vi "Prime BSI Camera Engine.vi"(0 "Prime Notifier Name":string="Not a Name", 11 "Camera Index":string[](array[string])) -> ()   [LabVIEW 2016]
uses:
  Prime BSI Controls/Prime Parameters.ctl
  Prime BSI Controls/Prime Parameter List.ctl
  Prime BSI Controls/Prime ROI.ctl
  Prime BSI Controls/Prime Notifier Element.ctl
  Prime BSI Controls/Prime Actions.ctl
  <vilib>/vision/Image Controls.llb/IMAQ Image.ctl
  Prime BSI Controls/Prime IMAQ Key Info.ctl
  TIFF Image Read and Write/TIF Write Image Information.ctl
  <vilib>/ptbypt/NI_PtbyPt.lvlib
panel:
  in  "Timing Mode":u32=1
  in  "Set Trigger":bool
  out "mean":dbl format="%0.2f"
  out "Value":dbl format="%.2f"
  in  "Parameter ID":u32
  out "fps":dbl
  out "Image Key Error":errorcluster
  out "Frame":u32
  in  "Init Camera":bool
  in  "Quit":bool
  in  "Use Display Module":bool
  in  "Capture":bool
  in  "Live Preview":bool
  in  "Get ROI":bool
  in  "Set ROI":bool
  in  "Get Parameter":bool
  in  "Set Parameter":bool
  in  "File Save Path":path
  in  "# of Frames":u32
  in  "ROI Setup":T1
  in  "Prime Parameter":T2
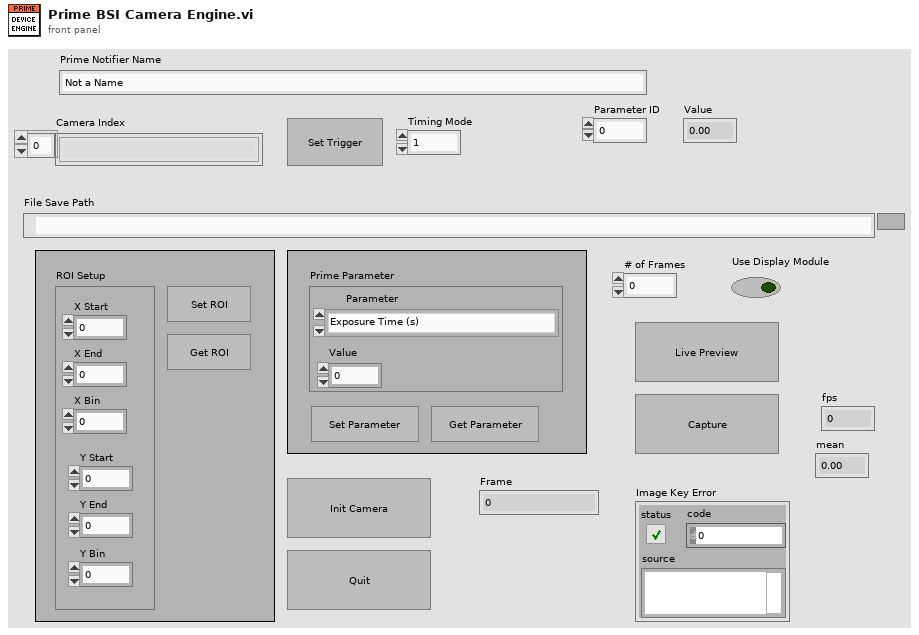
[diagram p1: front panel]
types:
  T1 = typedef "Prime ROI.ctl" = cluster{"X Start":u32, "X End":u32, "X Bin":u32, "Y Start":u32, "Y End":u32, "Y Bin":u32}
  T2 = typedef "Prime Parameters.ctl" = cluster{"Parameter":T3, "Value":dbl}
  T3 = typedef "Prime Parameter List.ctl" = enum16{"Exposure Time (s)"}
  T4 = typedef "Prime Actions.ctl" = enum16{"Error Check", "Initialize", "Preview", "Record", "Abort", "Record Settings", "Set Parameter", "Get Parameter", "Set ROI", "Get ROI", "Status", "Set Trigger", "Quit"}
  T5 = typedef "Image Type" = u32
  T6 = typedef "Prime Notifier Element.ctl" = cluster{"Prime Actions":T4, "Received?":bool, "Prime Parameter":T2, "Prime ROI":T1, "Running?":bool, "File Path":path, "# of frames":u32, "Image Ref":T7, "Error":errorcluster}
  T7 = typedef "IMAQ Image.ctl" = refnum<image>
  T8 = typedef "Prime IMAQ Key Info.ctl" = cluster{"Frame":u32, "Sensor Height":i32, "Sensor Width":i32, "ROI Height":i32, "ROI Width":i32, "ROI Enable?":bool, "Bit per Pixel":u8}
  T9 = enum32{"Invalid", "Standard", "Closed", "Hidden", "Minimized", "Maximized"}
  T10 = typedef "TIF Write Image Information.ctl" = cluster{"Image Width (Pixels)":u32, "Image Height (Pixels)":u32, "Pixel Width (µm)":dbl, "Pixel Height (µm)":dbl, "Bits Per Sample (e.g. 16)":u32, "No. of Frames":u32, "No. of Slices":u32, "Time Step (sec)":dbl, "Z Step (µm)":dbl}
  T11 = enum16{"big-endian, network order", "native, host order", "little-endian"}
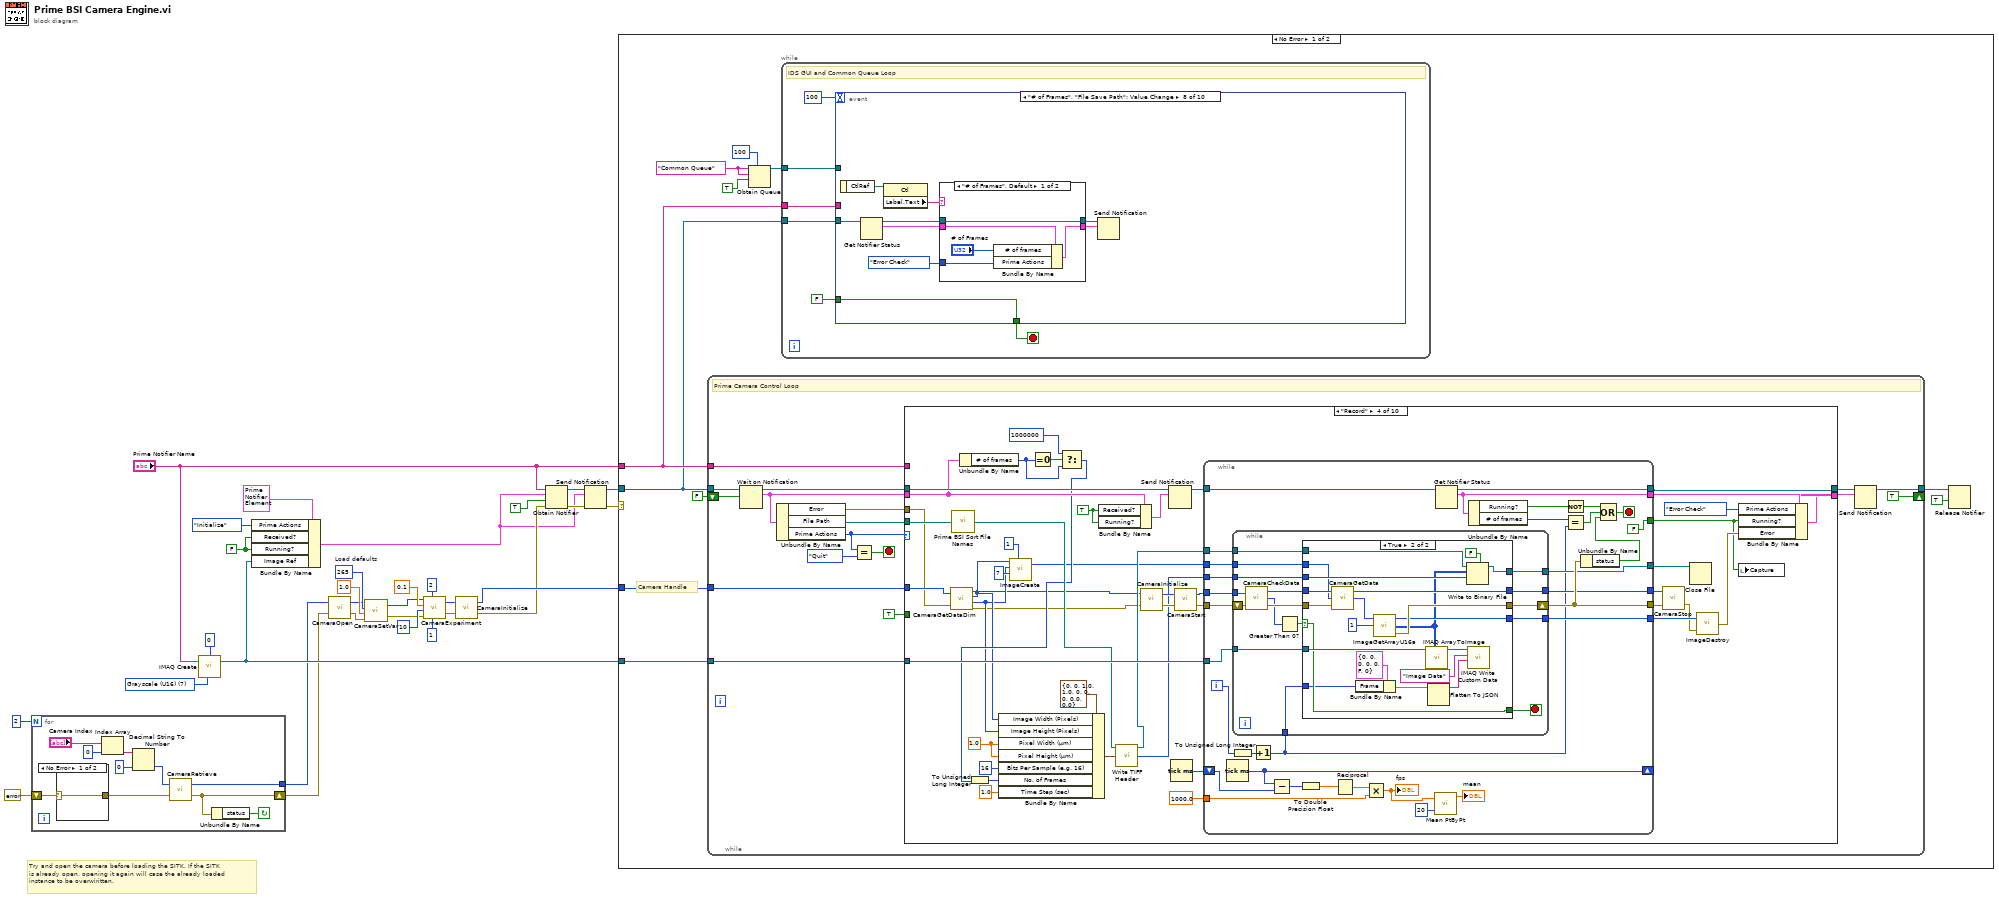
[diagram p0: block diagram]
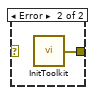
[diagram p2: hidden frame]
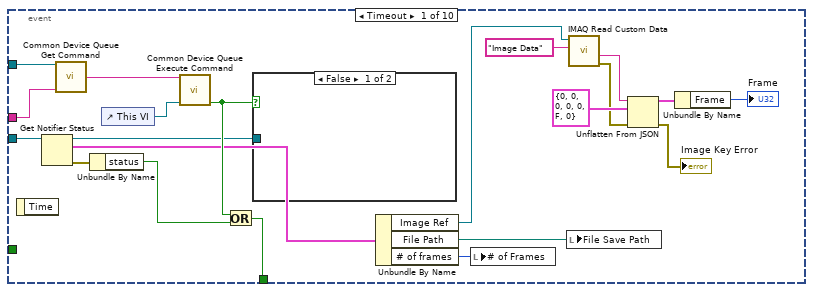
[diagram p3: hidden frame]
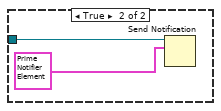
[diagram p4: hidden frame]
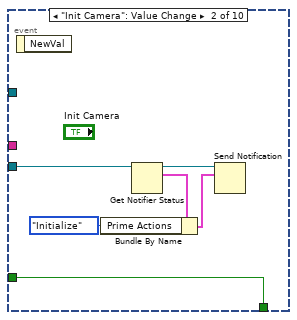
[diagram p5: hidden frame]
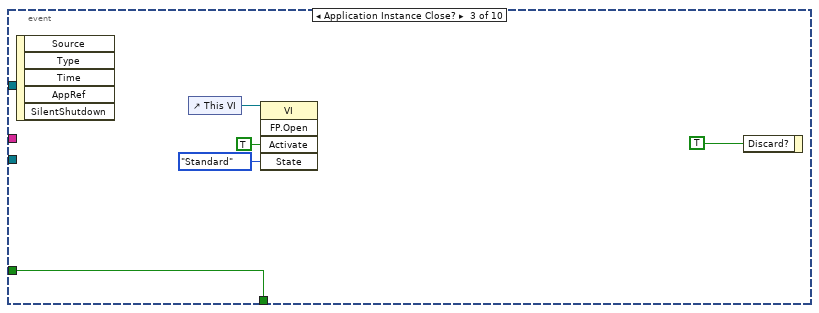
[diagram p6: hidden frame]
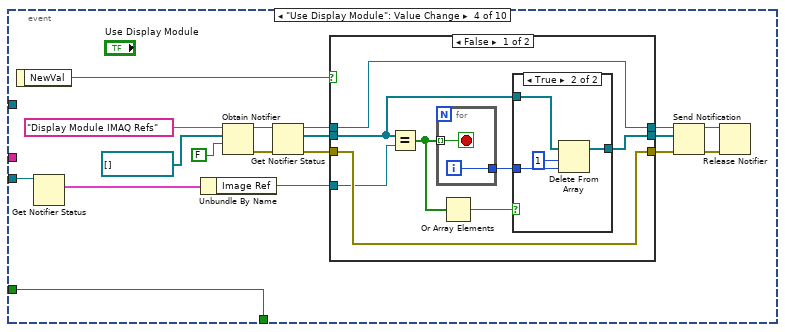
[diagram p7: hidden frame]
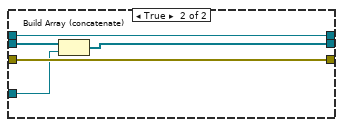
[diagram p9: hidden frame]
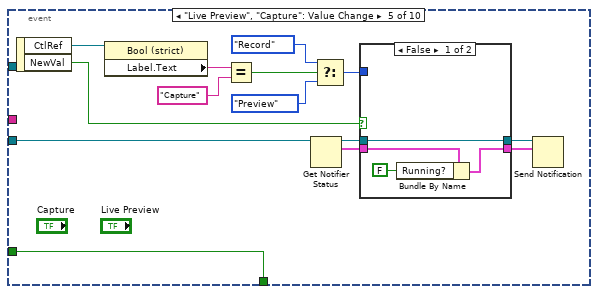
[diagram p10: hidden frame]
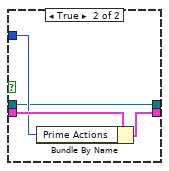
[diagram p11: hidden frame]
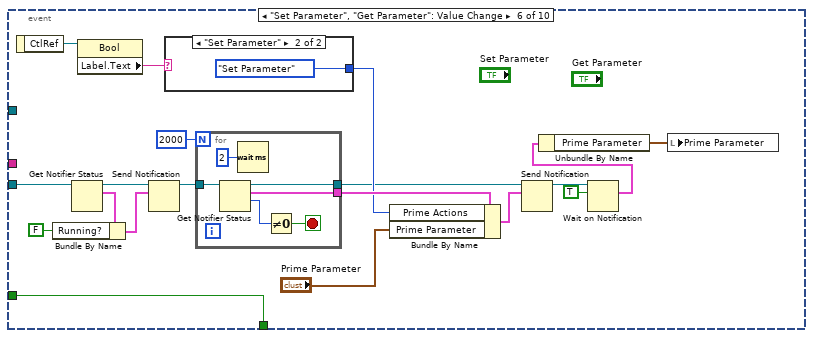
[diagram p12: hidden frame]
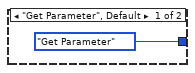
[diagram p13: hidden frame]
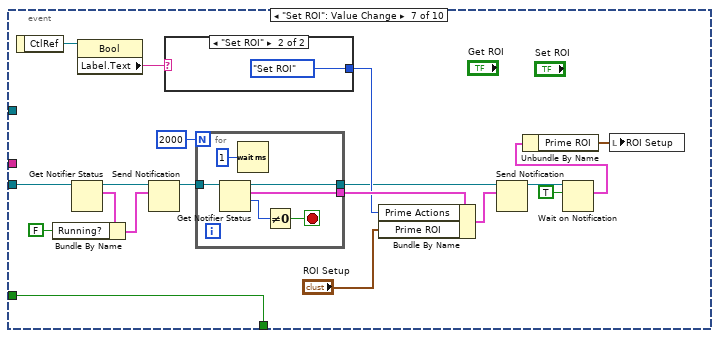
[diagram p14: hidden frame]
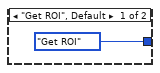
[diagram p15: hidden frame]
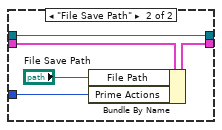
[diagram p16: hidden frame]
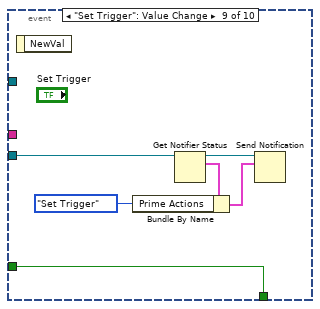
[diagram p17: hidden frame]
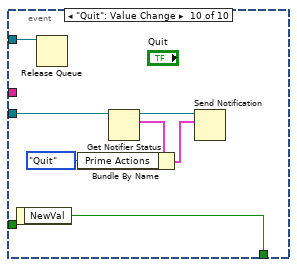
[diagram p18: hidden frame]
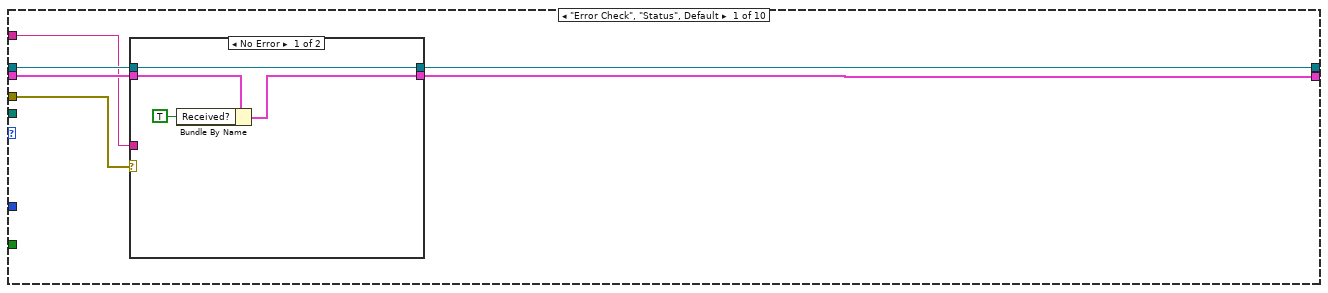
[diagram p19: hidden frame]
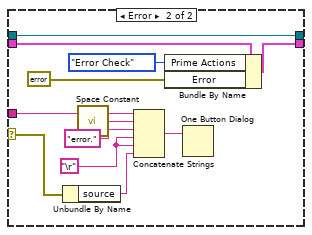
[diagram p20: hidden frame]
diagram:
  w19 = u32 265  # Load defaults
  w21 = FALSE ("Received?")
  w25 = T5 7 items=["Grayscale (U8)", "Grayscale (I16)", "Grayscale (SGL)", "Complex (CSG)", "RGB (U32)", "HSL (U32)", "RGB (U64)", "Grayscale (U16)"] ("Image Type")
  # "Try and open the camera before loading the SITK. If the SITK\nis already open, opening it again will case the already loaded\ninstance to be overwiritten."
  n1 = for {
    N: 2 -> [_]
    tunnel: [w36] -> w13
    shift-right: [w33] -> w12
    shift-left: errorcluster {"status"=FALSE, "code"=0, "source"=""} ("error out") -> [w35]
    stop <- w32 continue-if-true
    n2 = case shown="No Error" w35 {
      selector: w35 -> [w42 _]
      tunnel: [w42 w43] -> w34
      frame No Error {
      }
      frame Error {
        n3 = call <userlib>:"InitToolkit.vi"() -> ("error out"=w43:errorcluster)  [unwired: 1 in]
      }
    }
    n4 = Index Array(array="Camera Index", index=0) -> (element=w39:string)
    n5 = Decimal String To Number(string=w39, default (0L)=u32 0 ("default (0 I32)")) -> (number=w37:u32)  [unwired: 1 in, 1 out]
    n6 = call <userlib>:"CameraRetrieve.vi"("error in"=w34, "Camera Index"=w37) -> ("error out"=w33:errorcluster, "Device ID"=w36:u32)
    n7 = Unbundle By Name(w33) -> ("status"=w32:bool)
  }
  n8 = call "IMAQ Create"("Border Size"=0, "Image Name"="Prime Notifier Name", "Image Type"=w25) -> ("New Image"=w20:T7)  [unwired: 2 in, 1 out]
  n9 = Bundle By Name(cluster=T6 {"Prime Actions"=enum."Initialize", "Received?"=FALSE, "Prime Parameter"={"Parameter"=enum."Exposure Time (s)", "Value"=0.0}, "Prime ROI"={"X Start"=0, "X End"=0, "X Bin"=0, "Y Start"=0, "Y End"=0, "Y Bin"=0}, "Running?"=FALSE, "File Path"=path "", "# of frames"=0, "Image Ref"=refnum, "Error"={"status"=FALSE, "code"=0, "source"=""}} ("IDS Camera Cluster"), "Prime Actions"=Prime_Actions."Initialize" ("IDS Actions"), "Received?"=w21, "Running?"=w21, "Image Ref"=w20) -> (w1:T6)
  n10 = call <userlib>:"CameraOpen.vi"("error in"=w12, "Camera Device ID"=w13) -> ("error out"=w17:errorcluster, "Camera Handle"=w16:u32)
  n11 = call <userlib>:"CameraSetVar.vi"("error in"=w17, "Value"=1.0, "Parameter ID"=w19, "Camera Handle"=w16) -> ("error out"=w4:errorcluster, "CameraHandle"=w5:u32)
  n12 = call <userlib>:"CameraExperiment.vi"("Number of Accumulations"=u32 1, "Acquire / Focus Flag"=u32 2, "error in"=w4, "Number of Images"=u32 10 ("Acquire / Focus Flag"), "Exposure (sec)"=0.1, "Camera Handle"=w5) -> ("error out"=w10:errorcluster, "Camera Handle"=w11:u32)
  n13 = call <userlib>:"CameraInitialize.vi"("error in"=w10, "Camera Handle"=w11) -> ("error out"=w2:errorcluster, "Camera Handle"=w3:u32)
  n14 = Obtain Notifier(name (unnamed)="Prime Notifier Name", notification data type=w1, create if not found? (T)=TRUE, error in (no error)=w2) -> (notifier out=w30:refnum<notifier>, error out=w29:errorcluster)  [unwired: 1 out]
  n15 = Send Notification(notification=w1, notifier=w30, error in (no error)=w29) -> (notifier out=w28:refnum<notifier>, error out=w27:errorcluster)
  n16 = case shown="No Error" w27 {
    selector: w27 -> [_ w603]
    tunnel: w28 -> [w45 w604]
    tunnel: "Prime Notifier Name" -> [w46 w602]
    tunnel: w3 -> [w44 w593]
    tunnel: w20 -> [w52 w596]
    frame No Error {
      w50 = "Common Queue" ("Unique Notifier Name")
      # "Camera Handle"
      n17 = while {
        tunnel: w45 -> [w255]
        tunnel: [w256] -> w53
        tunnel: w44 -> [w249]
        tunnel: w52 -> [w248]
        tunnel: w46 -> [w244]
        shift-right: [TRUE] -> _
        shift-left: FALSE -> [w247]
        stop <- w257 stop-if-true
        # "Prime Camera Control Loop"
        n18 = Wait on Notification(notifier=w255, ignore previous (F)=w247) -> (notifier out=w254:refnum<notifier>, notification=w253:T6)  [unwired: 2 in, 2 out]
        n19 = Unbundle By Name(w253) -> ("Error"=w243:errorcluster, "File Path"=w241:path, "Prime Actions"=w252:T4)
        n20 = Equal?(x=w252, y=Prime_Actions."Quit") -> (x = y?=w257:bool)
        n21 = case shown="\"Record\"" w252 {
          tunnel: w254 -> [w263 w326 w355 w443 w518 w535 w547 w569 w582 w590]
          tunnel: [w262 w326 w334 w428 w518 w535 w547 w569 w582 w590] -> w250
          tunnel: w253 -> [w261 w325 w354 w417 w519 w533 w548 w570 w580 w589]
          tunnel: w244 -> [w260 _ _ _ _ _ _ _ _ _]
          tunnel: w249 -> [_ w312 w349 w438 w522 w530 w564 _ w576 w584]
          tunnel: w248 -> [_ w281 w340 w433 _ _ w551 _ _ w586]
          tunnel: [w259 w323 w353 w442 w525 w536 w566 w572 w578 w587] -> w246
          tunnel: TRUE -> [_ _ _ _ _ _ _ _ _ _]
          tunnel: w243 -> [w258 w280 w327 w398 w523 _ w546 w571 _ _]
          tunnel: w241 -> [_ _ _ w423 _ _ _ _ _ _]
          frame "Error Check", "Status", Default {
            n22 = case shown="No Error" w258 {
              selector: w258 -> [_ w270]
              tunnel: w261 -> [w266 w279]
              tunnel: [w267 w277] -> w262
              tunnel: w263 -> [w267 w277]
              tunnel: w260 -> [_ w276]
              tunnel: [w264 w272] -> w259
              frame No Error {
                n23 = Bundle By Name(cluster=w266, "Received?"=TRUE) -> (w264:T6)
              }
              frame Error {
                w271 = "\r"
                n24 = Unbundle By Name(w270) -> ("source"=w269:string)
                n25 = call <vilib>:"Space Constant.vi"() -> ("String"=w275:string)
                n26 = Concatenate Strings(w276, w275, "error." ("string"), w271, w271, w269) -> (w273:string)
                n27 = Bundle By Name(cluster=w279, "Prime Actions"=Prime_Actions."Error Check" ("IDS Actions"), "Error"=errorcluster {"status"=FALSE, "code"=0, "source"=""}) -> (w272:T6)
                n28 = One Button Dialog(message=w273) -> ()  [unwired: 1 in, 1 out]
              }
            }
          }
          frame "Initialize" {
            w287 = -2  # -2 = fastest adc
            w283 = -1  # -1 = keep what is currently set
            w291 = u32 1 items=["N/A", "Timed Mode/Free run", "Trigger First (only PM)", "Strobed/Ext Sync"] ("Timing Mode")
            w290 = u32 2  # Trigger Edge
            w295 = u32 3  # Shutter State
            w294 = u32 0  # Shutter Comp Time
            w299 = u32 1  # Number of Clears
            w298 = u32 50  # Number of Strips Per Clear
            w300 = u32 0  # Continuous Clears
            w282 = u32 2048 ("X End")
            w304 = u32 1 ("X Start")
            w306 = u32 1  # ROI Number
            w309 = u32 2 items=["Never", "Pre Expos", "Pre Seq", "Post Seq", "Pre-Post Seq", "Pre Expos, Post Seq"] ("Clear Mode")
            w310 = u32 32  # Clear Mode
            w313 = u32 0 items=["First Row", "All Rows", "Any Row", "Max Exposure"] ("Exposure Out")
            w315 = u32 255  # Exposure Out
            n29 = To Double Precision Float(number=w313) -> (double precision float=w314:dbl)
            n30 = call <userlib>:"CameraSetVar.vi"("error in"=w280, "Value"=w314, "Parameter ID"=w315, "Camera Handle"=w312) -> ("error out"=w307:errorcluster, "CameraHandle"=w308:u32)
            n31 = To Double Precision Float(number=w309) -> (double precision float=w311:dbl)
            n32 = Bundle By Name(cluster=T1 {"X Start"=0, "X End"=0, "X Bin"=0, "Y Start"=0, "Y End"=0, "Y Bin"=0} ("ROI Setup"), "X Start"=w304, "X End"=w282, "X Bin"=w304, "Y Start"=w304, "Y End"=w282, "Y Bin"=w304) -> (w303:T1)
            n33 = call <userlib>:"CameraSetVar.vi"("error in"=w307, "Value"=w311, "Parameter ID"=w310, "Camera Handle"=w308) -> ("error out"=w301:errorcluster, "CameraHandle"=w302:u32)
            n34 = call <userlib>:"CameraROI.vi"("error in"=w301, "ROI Params"=w303, "ROI Index"=w306, "Camera Handle"=w302) -> ("error out"=w296:errorcluster, "Camera Handle"=w297:u32)
            n35 = Bundle By Name(cluster=T8 {"Frame"=0, "Sensor Height"=0, "Sensor Width"=0, "ROI Height"=0, "ROI Width"=0, "ROI Enable?"=FALSE, "Bit per Pixel"=0} ("IDS IMAQ Key Info"), "Frame"=u32 0, "Sensor Height"=w282, "Sensor Width"=w282, "ROI Height"=w282, "ROI Width"=w282, "ROI Enable?"=FALSE, "Bit per Pixel"=u8 16) -> (w320:T8)
            n36 = call <userlib>:"CameraCleans.vi"("Camera Handle"=w297, "Number of Clears"=w299, "Number of Strips Per Clear"=w298, "error in"=w296, "Continuous Clears"=w300) -> ("Camera Handle"=w293:u32, "error out"=w292:errorcluster)
            n37 = call <userlib>:"CameraShutter.vi"("Camera Handle"=w293, "Shutter Comp Time: Pre Open"=w294, "Shutter Comp Time: Post Open"=w294, "error in"=w292, "Shutter State"=w295) -> ("Camera Handle"=w289:u32, "error out"=w288:errorcluster)
            n38 = Flatten To JSON(anything=w320) -> (JSON string=w322:string)  [unwired: 2 in, 1 out]
            n39 = call <userlib>:"CameraTrigger.vi"("error in"=w288, "Trigger Edge"=w290, "Timing Mode"=w291, "Camera Handle"=w289) -> ("error out"=w285:errorcluster, "Camera Handle"=w286:u32)
            n40 = call "IMAQ Write Custom Data"("Custom Data In"=w322, "Key"="Image Data", "Image"=w281) -> ()  [unwired: 7 in, 2 out]
            n41 = call <userlib>:"CameraADCset.vi"("ADC offset"=w283, "Read Out port"=w283, "error in (no error)"=w285, "ADC Gain"=w283, "ADC Speed"=w287, "Camera Handle"=w286) -> ("error out"=w284:errorcluster)  [unwired: 1 out]
            n42 = Bundle By Name(cluster=w325, "Prime Actions"=Prime_Actions."Error Check" ("IDS Actions"), "Error"=w284) -> (w323:T6)
          }
          frame "Preview" {
            w331 = FALSE ("Running?")
            w351 = TRUE ("Received?")
            n43 = Bundle By Name(cluster=w354, "Received?"=w351, "Running?"=w351) -> (w352:T6)
            n44 = call <userlib>:"CameraGetDataDim.vi"("Camera Handle"=w349, "error in"=w327) -> ("Camera Handle"=w329:u32, "Xdim"=w348:u32, "Ydim"=w347:u32, "error out"=w344:errorcluster)
            n45 = call <userlib>:"ImageCreate.vi"("X dimension"=w348, "Y dimension"=w347, "Data Type"=u32 7, "error in"=w344, "Number Of Frames"=u32 1) -> ("Image Handle"=w343:u32, "error out"=w328:errorcluster)
            n46 = Send Notification(notification=w352, notifier=w355) -> (notifier out=w339:refnum<notifier>)  [unwired: 1 in, 1 out]
            n47 = call <userlib>:"CameraStart.vi"("error in"=w328, "Camera Handle"=w329) -> ("error out"=w341:errorcluster, "Camera Handle"=w342:u32)
            n48 = while {
              tunnel: w342 -> [w375]
              tunnel: w341 -> [w374]
              tunnel: w343 -> [w371]
              tunnel: w339 -> [w361]
              tunnel: [w360] -> w334
              tunnel: [w363] -> w336
              tunnel: [w373] -> w337
              tunnel: [w372] -> w335
              tunnel: w340 -> [w370]
              tunnel: [w358] -> w333
              shift-right: [w356] -> _
              shift-left: u32 0 ("Frame") -> [w357]
              stop <- w369 stop-if-true
              n49 = call <userlib>:"CameraCheckData.vi"("Camera Handle"=w375, "error in"=w374) -> ("Camera Handle"=w367:u32, "Number Of Frames Available"=w365:i32, "error out"=w368:errorcluster)
              n50 = Greater Than 0?(x=w365) -> (x > 0?=w366:bool)
              n51 = case shown="True" w366 {
                tunnel: w371 -> [w377 w394]
                tunnel: w368 -> [w379 w392]
                tunnel: [w379 w397] -> w363
                tunnel: [w377 w396] -> w372
                tunnel: [w378 w390] -> w373
                tunnel: w367 -> [w378 w393]
                tunnel: w370 -> [_ w387]
                tunnel: w357 -> [w376 w381]
                tunnel: [w376 w380] -> w356
                frame False {
                }
                frame True {
                  n52 = Increment(x=w381) -> (x+1=w380:u32)
                  n53 = call <userlib>:"CameraGetData.vi"("error in"=w392, "Image/Data Handle"=w394, "Camera Handle"=w393) -> ("error out"=w389:errorcluster, "Image/Data Handle"=w391:u32, "Camera Handle"=w390:u32)
                  n54 = Bundle By Name(cluster=T8 {"Frame"=0, "Sensor Height"=0, "Sensor Width"=0, "ROI Height"=0, "ROI Width"=0, "ROI Enable?"=FALSE, "Bit per Pixel"=0} ("IDS IMAQ Key Info"), "Frame"=w380) -> (w383:T8)
                  n55 = call <userlib>:"ImageGetArrayU16a.vi"("error in"=w389, "Z position"=u32 1, "Data Handle"=w391) -> ("error out"=w397:errorcluster, "Array uint 16"=w388:u16[][], "Data Handle"=w396:u32)  [unwired: 1 in]
                  n56 = call "IMAQ ArrayToImage"("Image Pixels (U16)"=w388, "Image"=w387) -> ("Image Out"=w382:T7)  [unwired: 8 in, 1 out]
                  n57 = Flatten To JSON(anything=w383) -> (JSON string=w385:string)  [unwired: 2 in, 1 out]
                  n58 = call "IMAQ Write Custom Data"("Custom Data In"=w385, "Key"="Image Data", "Image"=w382) -> ()  [unwired: 7 in, 2 out]
                }
              }
              n59 = Get Notifier Status(notifier=w361) -> (notifier out=w360:refnum<notifier>, current notification=w358:T6)  [unwired: 1 in, 3 out]
              n60 = Unbundle By Name(w358) -> ("Running?"=w362:bool)
              n61 = Unbundle By Name(w363) -> ("status"=w364:bool)
              n62 = Not(x=w362) -> (.not. x?=w359:bool)
              n63 = Or(x=w359, y=w364) -> (x .or. y?=w369:bool)
            }
            n64 = call <userlib>:"CameraStop.vi"("error in"=w336, "Camera Handle"=w337) -> ("error out"=w338:errorcluster)  [unwired: 1 out]
            n65 = call <userlib>:"ImageDestroy.vi"("error in"=w338, "Data handle"=w335) -> ("error out"=w332:errorcluster)
            n66 = Bundle By Name(cluster=w333, "Prime Actions"=Prime_Actions."Error Check", "Running?"=w331, "Error"=w332) -> (w353:T6)
            n67 = local write "Capture"(w331) -> ()
          }
          frame "Record" {
            w420 = 1.0 ("Pixel Width (µm)")
            w440 = TRUE ("Received?")
            n68 = call <userlib>:"CameraGetDataDim.vi"("Camera Handle"=w438, "error in"=w398) -> ("Camera Handle"=w400:u32, "Xdim"=w406:u32, "Ydim"=w405:u32, "error out"=w399:errorcluster)
            n69 = call "Prime BSI Sort File Names.vi"("Requested File Path"=w423) -> ("Resulting File Path"=w418:path)  [unwired: 14 in]
            n70 = Unbundle By Name(w417) -> ("# of frames"=w415:u32)
            n71 = call <userlib>:"ImageCreate.vi"("X dimension"=w406, "Y dimension"=w405, "Data Type"=u32 7, "Number Of Frames"=u32 1) -> ("Image Handle"=w404:u32)  [unwired: 1 in, 1 out]
            n72 = Equal To 0?(x=w415) -> (x = 0?=w416:bool)
            n73 = Select(t=1000000, s=w416, f=w415) -> (s? t:f=w413:u32)
            n74 = To Unsigned Long Integer(number=w413) -> (unsigned 32bit integer=w403:u32)
            n75 = Bundle By Name(cluster=T10 {"Image Width (Pixels)"=0, "Image Height (Pixels)"=0, "Pixel Width (µm)"=1.0, "Pixel Height (µm)"=1.0, "Bits Per Sample (e.g. 16)"=0, "No. of Frames"=0, "No. of Slices"=0, "Time Step (sec)"=0.0, "Z Step (µm)"=0.0} ("Image Info"), "Image Width (Pixels)"=w406, "Image Height (Pixels)"=w405, "Pixel Width (µm)"=w420, "Pixel Height (µm)"=w420, "Bits Per Sample (e.g. 16)"=u32 16, "No. of Frames"=w403, "Time Step (sec)"=1.0) -> (w422:T10)
            n76 = Bundle By Name(cluster=w417, "Received?"=w440, "Running?"=w440) -> (w441:T6)
            n77 = call "Write TIFF Header.vi"("File Path"=w418, "Image Info"=w422) -> ("File Ref"=w411:refnum<file>, "Byte Order"=w410:T11)  [unwired: 11 in, 1 out]
            n78 = call <userlib>:"CameraInitialize.vi"("error in"=w399, "Camera Handle"=w400) -> ("error out"=w437:errorcluster, "Camera Handle"=w436:u32)
            n79 = Send Notification(notification=w441, notifier=w443) -> (notifier out=w432:refnum<notifier>)  [unwired: 1 in, 1 out]
            n80 = Tick Count (ms)() -> (millisecond timer value=w425:u32)
            n81 = call <userlib>:"CameraStart.vi"("error in"=w437, "Camera Handle"=w436) -> ("error out"=w434:errorcluster, "Camera Handle"=w435:u32)
            n82 = while {
              tunnel: w435 -> [w475]
              tunnel: w434 -> [w474]
              tunnel: w432 -> [w473]
              tunnel: [w472] -> w428
              tunnel: [w469] -> w430
              tunnel: [w468] -> w431
              tunnel: [w467] -> w429
              tunnel: w433 -> [w465]
              tunnel: [w464] -> w427
              shift-right: [w458] -> _
              shift-left: w425 -> [w459]
              tunnel: 1000.0 -> [w454]
              tunnel: w411 -> [w453]
              tunnel: w410 -> [w452]
              tunnel: [w451] -> w409
              tunnel: w404 -> [w450]
              tunnel: [FALSE ("Running?")] -> w402
              i -> [w462]
              stop <- w470 stop-if-true
              n83 = Tick Count (ms)() -> (millisecond timer value=w458:u32)
              n84 = To Unsigned Long Integer(number=w462) -> (unsigned 32bit integer=w444:u32)
              n85 = Increment(x=w444) -> (x+1=w448:u32)
              n86 = while {
                tunnel: w475 -> [w491]
                tunnel: [w486] -> w468
                tunnel: [w485] -> w467
                tunnel: w465 -> [w482]
                shift-right: [w488] -> w469
                shift-left: w474 -> [w490]
                tunnel: w453 -> [w480]
                tunnel: w452 -> [w479]
                tunnel: [w478] -> w451
                tunnel: w450 -> [w477]
                tunnel: w448 -> [w476]
                stop <- w481 stop-if-true
                n87 = call <userlib>:"CameraCheckData.vi"("Camera Handle"=w491, "error in"=w490) -> ("Camera Handle"=w487:u32, "Number Of Frames Available"=w484:i32, "error out"=w489:errorcluster)
                n88 = Greater Than 0?(x=w484) -> (x > 0?=w483:bool)
                n89 = case shown="True" w483 {
                  selector: w483 -> [w494 w505]
                  tunnel: w489 -> [w496 w513]
                  tunnel: [w496 w517] -> w488
                  tunnel: [w492 w516] -> w485
                  tunnel: [w495 w512] -> w486
                  tunnel: w487 -> [w495 w514]
                  tunnel: w482 -> [_ w511]
                  tunnel: w476 -> [_ w497]
                  tunnel: [w494 w505] -> w481
                  tunnel: w480 -> [w493 w502]
                  tunnel: w479 -> [_ w501]
                  tunnel: [w493 w499] -> w478
                  tunnel: w477 -> [w492 w498]
                  frame False {
                  }
                  frame True {
                    n90 = call <userlib>:"CameraGetData.vi"("error in"=w513, "Image/Data Handle"=w498, "Camera Handle"=w514) -> ("Image/Data Handle"=w504:u32, "Camera Handle"=w512:u32)  [unwired: 1 out]
                    n91 = Bundle By Name(cluster=T8 {"Frame"=0, "Sensor Height"=0, "Sensor Width"=0, "ROI Height"=0, "ROI Width"=0, "ROI Enable?"=FALSE, "Bit per Pixel"=0} ("IDS IMAQ Key Info"), "Frame"=w497) -> (w507:T8)
                    n92 = call <userlib>:"ImageGetArrayU16a.vi"("Z position"=u32 1, "Data Handle"=w504) -> ("error out"=w517:errorcluster, "Array uint 16"=w500:u16[][], "Data Handle"=w516:u32)  [unwired: 2 in]
                    n93 = call "IMAQ ArrayToImage"("Image Pixels (U16)"=w500, "Image"=w511) -> ("Image Out"=w506:T7)  [unwired: 8 in, 1 out]
                    n94 = Flatten To JSON(anything=w507) -> (JSON string=w509:string)  [unwired: 2 in, 1 out]
                    n95 = Write to Binary File(file (use dialog)=w502, data=w500, 5:FALSE ("prepend array or string size? (T)"), 9:w501) -> (refnum out=w499:refnum<file>)  [unwired: 2 in, 2 out]
                    n96 = call "IMAQ Write Custom Data"("Custom Data In"=w509, "Key"="Image Data", "Image"=w506) -> ()  [unwired: 7 in, 2 out]
                  }
                }
              }
              n97 = Subtract(x=w458, y=w459) -> (x-y=w457:u32)
              n98 = To Double Precision Float(number=w457) -> (double precision float=w456:dbl)
              n99 = Reciprocal(x=w456) -> (1/x=w455:dbl)
              n100 = Multiply(x=w455, y=w454) -> (x*y=w447:dbl)
              "fps" <- w447
              n101 = call <vilib>:"Mean PtByPt.vi"("x"=w447, "sample length"=20) -> ("mean"=→"mean":dbl)  [unwired: 2 in, 1 out]
              n102 = Get Notifier Status(notifier=w473) -> (notifier out=w472:refnum<notifier>, current notification=w464:T6)  [unwired: 1 in, 3 out]
              n103 = Unbundle By Name(w464) -> ("Running?"=w471:bool, "# of frames"=w463:u32)
              n104 = Not(x=w471) -> (.not. x?=w466:bool)
              n105 = Equal?(x=w463, y=w448) -> (x = y?=w461:bool)
              n106 = Unbundle By Name(w469) -> ("status"=w460:bool)
              n107 = Compound Arithmetic op=OR(w466, w461, w460) -> (w470:bool)
            }
            n108 = call <userlib>:"CameraStop.vi"("error in"=w430, "Camera Handle"=w431) -> ("error out"=w412:errorcluster)  [unwired: 1 out]
            n109 = Close File(refnum=w409) -> ()  [unwired: 1 in, 2 out]
            n110 = call <userlib>:"ImageDestroy.vi"("error in"=w412, "Data handle"=w429) -> ("error out"=w426:errorcluster)
            n111 = Bundle By Name(cluster=w427, "Prime Actions"=Prime_Actions."Error Check", "Running?"=w402, "Error"=w426) -> (w442:T6)
            n112 = local write "Capture"(w402) -> ()
          }
          frame "Get Parameter" {
            n113 = call <userlib>:"CameraGetVar.vi"("Parameter ID"="Parameter ID", "Camera Handle"=w522) -> ("Value"=→"Value":dbl)  [unwired: 1 in, 2 out]
            n114 = Bundle By Name(cluster=w519, "Prime Actions"=Prime_Actions."Error Check" ("IDS Actions"), "Error"=w523, "Received?"=TRUE) -> (w525:T6)
          }
          frame "Set Parameter" {
            n115 = Unbundle By Name(w533) -> ("Prime Parameter.Parameter"=w532:T3, "Prime Parameter.Value"=w531:dbl)
            n116 = case shown="\"Exposure Time (s)\", Default" w532 {
              tunnel: w531 -> [w541]
              tunnel: [w540] -> w529
              tunnel: w530 -> [w539]
              tunnel: [w538] -> w528
              frame "Exposure Time (s)", Default {
                n117 = call <userlib>:"CameraExperiment.vi"("Number of Accumulations"=u32 1, "Acquire / Focus Flag"=u32 2, "Number of Images"=u32 10 ("Acquire / Focus Flag"), "Exposure (sec)"=w541, "Camera Handle"=w539) -> ("error out"=w540:errorcluster, "Camera Handle"=w538:u32)  [unwired: 1 in]
              }
            }
            n118 = call <userlib>:"CameraInitialize.vi"("error in"=w529, "Camera Handle"=w528) -> ("error out"=w527:errorcluster)  [unwired: 1 out]
            n119 = Bundle By Name(cluster=w533, "Prime Actions"=Prime_Actions."Error Check" ("IDS Actions"), "Received?"=TRUE, "Error"=w527) -> (w536:T6)
          }
          frame "Set ROI" {
            w552 = "Image Data" ("Key")
            n120 = Unbundle By Name(w548) -> ("Prime ROI"=w563:T1)
            n121 = call <userlib>:"CameraROI.vi"("error in"=w546, "ROI Params"=w563, "ROI Index"=u32 1, "Camera Handle"=w564) -> ("error out"=w561:errorcluster, "Camera Handle"=w562:u32)
            n122 = call <userlib>:"CameraGetDataDim.vi"("Camera Handle"=w562, "error in"=w561) -> ("Xdim"=w550:u32, "Ydim"=w549:u32, "error out"=w545:errorcluster)  [unwired: 1 out]
            n123 = Bundle By Name(cluster=w548, "Prime Actions"=Prime_Actions."Error Check" ("IDS Actions"), "Error"=w545, "Received?"=TRUE) -> (w566:T6)
            n124 = call "IMAQ Read Custom Data"("Key"=w552, "Image"=w551) -> ("Custom Data Out"=w559:string, "Image (duplicate)"=w560:T7)  [unwired: 7 in, 1 out]
            n125 = To Long Integer(number=w550) -> (32bit integer=w554:i32)
            n126 = To Long Integer(number=w549) -> (32bit integer=w553:i32)
            n127 = Unflatten From JSON(JSON string=w559, type and defaults=T8 {"Frame"=0, "Sensor Height"=0, "Sensor Width"=0, "ROI Height"=0, "ROI Width"=0, "ROI Enable?"=FALSE, "Bit per Pixel"=0} ("IDS IMAQ Key Info")) -> (value=w558:T8)  [unwired: 5 in, 1 out]
            n128 = Bundle By Name(cluster=w558, "ROI Width"=w554, "ROI Height"=w553) -> (w556:T8)
            n129 = Flatten To JSON(anything=w556) -> (JSON string=w555:string)  [unwired: 2 in, 1 out]
            n130 = call "IMAQ Write Custom Data"("Custom Data In"=w555, "Key"=w552, "Image"=w560) -> ()  [unwired: 7 in, 2 out]
          }
          frame "Get ROI" {
            n131 = Bundle By Name(cluster=w570, "Prime Actions"=Prime_Actions."Error Check" ("IDS Actions"), "Error"=w571, "Received?"=TRUE) -> (w572:T6)
          }
          frame "Set Trigger" {
            # "1: Positive Edge\n2: Negative Edge"
            # "Timing Mode\n\n1 = No external trigger (trigger is internal to camera)\n\n2 = External trigger activates all data collection\n\n3 = Each exposure requires a trigger\n\n4 = An external trigger signal controls both the beginning and end of each exposure (Bulb mode). This mode is not valid for all cameras.\n\n5 = External triggers may occur at uneven intervals (Variable mode). This mode is not valid for all cameras.\n\n6 = External trigger activates all data collection (Flash mode). In addition, if the camera is fitted with a flash port, the signal is brought out to these pins. This mode is not valid for all cameras.\n\n7 = Internal trigger. For use when triggering is controlled by a pulse timing generator such as the Princeton Instruments PTG. Note that this mode does not work with older PTG systems."
            n132 = Bundle By Name(cluster=w580, "Prime Actions"=Prime_Actions."Set Trigger", "Received?"=TRUE) -> (w578:T6)
            n133 = call <userlib>:"CameraTrigger.vi"("Trigger Edge"=u32 1, "Timing Mode"="Timing Mode", "Camera Handle"=w576) -> ()  [unwired: 1 in, 2 out]
          }
          frame "Quit" {
            n134 = call "IMAQ Dispose"("Image"=w586) -> ()  [unwired: 5 in, 1 out]
            n135 = call <userlib>:"CameraClose.vi"("Camera Handle"=w584) -> ("error out"=w585:errorcluster)  [unwired: 1 in]
            n136 = call <userlib>:"UninitToolkit.vi"("error in"=w585) -> ("error out"=w583:errorcluster)
            n137 = Bundle By Name(cluster=w589, "Received?"=TRUE, "Error"=w583) -> (w587:T6)
          }
        }
        n138 = Send Notification(notification=w246, notifier=w250) -> (notifier out=w256:refnum<notifier>)  [unwired: 1 in, 1 out]
      }
      n139 = Obtain Queue(max queue size (-1, unlimited)=100, name (unnamed)=w50, element data type=w50, create if not found? (T)=TRUE) -> (queue out=w47:refnum<queue>)  [unwired: 1 in, 2 out]
      n140 = while {
        tunnel: w47 -> [w59]
        tunnel: w46 -> [w57]
        tunnel: w45 -> [w58]
        stop <- w56 stop-if-true
        # "IDS GUI and Common Queue Loop"
        n141 = event shown="[7] \"# of Frames\", \"File Save Path\": Value Change" {
          selector: _ -> [_ _ _ _ _ _ _ _ _ _]
          dyn-events: _ -> [_ _ _ _ _ _ _ _ _ _]
          timeout: 100 -> [_ _ _ _ _ _ _ _ _ _]
          tunnel: w59 -> [w75 _ _ _ _ _ _ _ _ w240]
          tunnel: w58 -> [w74 w88 _ w112 w137 w171 w198 w215 w232 w239]
          tunnel: w57 -> [w73 _ _ _ _ _ _ _ _ _]
          tunnel: [w72 w89 w94 w95 w146 w173 w200 w217 w233 w234] -> w56
          tunnel: FALSE -> [_ w89 w94 w95 w146 w173 w200 w217 w233 _]
          event Timeout {
            n142 = event-data() -> ()  [unwired: 1 in, 1 out]
            n143 = Get Notifier Status(notifier=w74) -> (notifier out=w76:refnum<notifier>, current notification=w69:T6, error out=w81:errorcluster)  [unwired: 1 in, 2 out]
            n144 = call "Common Device Queue Get Command.vi"("Common Queue"=w75, "Notifier Name"=w73) -> ("Command"=w80:string)  [unwired: 12 in, 1 out]
            n145 = Unbundle By Name(w81) -> ("status"=w78:bool)
            n146 = control-ref of="This VI"() -> (w79:refnum<vi>)
            n147 = call "Common Device Queue Execute Command.vi"("Common Command"=w80, "VI Refnum"=w79) -> ("Quit?"=w77:bool)  [unwired: 12 in, 1 out]
            n148 = Or(x=w77, y=w78) -> (x .or. y?=w72:bool)
            n149 = case shown="False" w77 {
              tunnel: w76 -> [_ w83]
              frame False {
              }
              frame True {
                n150 = Send Notification(notification=T6 {"Prime Actions"=enum."Quit", "Received?"=FALSE, "Prime Parameter"={"Parameter"=enum."Exposure Time (s)", "Value"=0.0}, "Prime ROI"={"X Start"=0, "X End"=0, "X Bin"=0, "Y Start"=0, "Y End"=0, "Y Bin"=0}, "Running?"=FALSE, "File Path"=path "", "# of frames"=0, "Image Ref"=refnum, "Error"={"status"=FALSE, "code"=0, "source"=""}} ("IDS Camera Cluster"), notifier=w83) -> ()  [unwired: 1 in, 2 out]
              }
            }
            n151 = Unbundle By Name(w69) -> ("Image Ref"=w67:T7, "File Path"=w71:path, "# of frames"=w70:u32)
            n152 = local write "# of Frames"(w70) -> ()
            n153 = local write "File Save Path"(w71) -> ()
            n154 = call "IMAQ Read Custom Data"("Key"="Image Data", "Image"=w67) -> ("error out"=w62:errorcluster, "Custom Data Out"=w65:string)  [unwired: 7 in, 1 out]
            n155 = Unflatten From JSON(JSON string=w65, type and defaults=T8 {"Frame"=0, "Sensor Height"=0, "Sensor Width"=0, "ROI Height"=0, "ROI Width"=0, "ROI Enable?"=FALSE, "Bit per Pixel"=0} ("IDS IMAQ Key Info"), error in (no error)=w62) -> (value=w64:T8, error out=→"Image Key Error":errorcluster)  [unwired: 4 in]
            n156 = Unbundle By Name(w64) -> ("Frame"=→"Frame":u32)
          }
          event "Init Camera": Value Change {
            n157 = event-data() -> ()  [unwired: 1 in, 1 out]
            n158 = Get Notifier Status(notifier=w88) -> (notifier out=w84:refnum<notifier>, current notification=w87:T6)  [unwired: 1 in, 3 out]
            n159 = Bundle By Name(cluster=w87, "Prime Actions"=Prime_Actions."Initialize" ("IDS Actions")) -> (w85:T6)
            n160 = Send Notification(notification=w85, notifier=w84) -> ()  [unwired: 1 in, 2 out]
          }
          event Application Instance Close? {
            n161 = event-data() -> ()  [unwired: 1 in, 5 out]
            n162 = control-ref of="This VI"() -> (w91:refnum<vi>)
            n163 = invoke class="VI" method="FP.Open"(reference=w91, "Activate"=TRUE ("Activate?"), "State"=T9."Standard") -> ()  [unwired: 2 in, 5 out]
            n164 = event-data("Discard?"=TRUE) -> ()  [unwired: 1 in, 1 out]
          }
          event "Use Display Module": Value Change {
            n165 = event-data() -> ("NewVal"=w97:bool)  [unwired: 1 in]
            n166 = Get Notifier Status(notifier=w112) -> (current notification=w111:T6)  [unwired: 1 in, 4 out]
            n167 = Unbundle By Name(w111) -> ("Image Ref"=w96:T7)
            n168 = Obtain Notifier(name (unnamed)="Display Module IMAQ Refs", notification data type=T7[] [], create if not found? (T)=FALSE) -> (notifier out=w104:refnum<notifier>, error out=w103:errorcluster)  [unwired: 1 in, 1 out]
            n169 = Get Notifier Status(notifier=w104, error in (no error)=w103) -> (notifier out=w105:refnum<notifier>, current notification=w107:T7[], error out=w106:errorcluster)  [unwired: 2 out]
            n170 = case shown="False" w97 {
              tunnel: w105 -> [w120 w130]
              tunnel: w106 -> [w114 w129]
              tunnel: w107 -> [w116 w132]
              tunnel: [w115 w131] -> w110
              tunnel: [w120 w130] -> w108
              tunnel: [w114 w129] -> w109
              tunnel: w96 -> [w113 w128]
              frame False {
                n171 = Equal?(x=w116, y=w113) -> (x = y?=w119:bool[])
                n172 = for {
                  tunnel: w119 -> [w127] mode=indexing
                  tunnel: [w126] -> w117
                  i -> [w126]
                  stop <- w127 stop-if-true
                }
                n173 = Or Array Elements(Boolean array=w119) -> (logical OR=w118:bool)
                n174 = case shown="True" w118 {
                  tunnel: w117 -> [_ w124]
                  tunnel: w116 -> [w121 w123]
                  tunnel: [w121 w122] -> w115
                  frame False {
                  }
                  frame True {
                    n175 = Delete From Array(array=w123, length=1, index=w124) -> (array with subset deleted=w122:T7[])  [unwired: 1 out]
                  }
                }
              }
              frame True {
                n176 = Build Array (concatenate)(w132, w128) -> (w131:T7[])
              }
            }
            n177 = Send Notification(notification=w110, notifier=w108, error in (no error)=w109) -> (notifier out=w102:refnum<notifier>, error out=w101:errorcluster)
            n178 = Release Notifier(notifier=w102, error in (no error)=w101) -> ()  [unwired: 1 in, 3 out]
          }
          event "Live Preview", "Capture": Value Change {
            n179 = event-data() -> ("CtlRef"=w145:refnum<vi>, "NewVal"=w139:bool)  [unwired: 1 in]
            n180 = property class="Bool (strict)"(reference=w145) -> ("Label.Text"=w144:string)  [unwired: 1 in, 2 out]
            n181 = Equal?(x=w144, y="Capture") -> (x = y?=w142:bool)
            n182 = Get Notifier Status(notifier=w137) -> (notifier out=w136:refnum<notifier>, current notification=w135:T6)  [unwired: 1 in, 3 out]
            n183 = Select(t=Prime_Actions."Record" ("y"), s=w142, f=Prime_Actions."Preview" ("y")) -> (s? t:f=w138:T4)
            n184 = case shown="False" w139 {
              tunnel: w138 -> [_ w153]
              tunnel: w136 -> [w148 w152]
              tunnel: w135 -> [w150 w154]
              tunnel: [w148 w152] -> w134
              tunnel: [w147 w151] -> w133
              frame False {
                n185 = Bundle By Name(cluster=w150, "Running?"=FALSE) -> (w147:T6)
              }
              frame True {
                n186 = Bundle By Name(cluster=w154, "Prime Actions"=w153) -> (w151:T6)
              }
            }
            n187 = Send Notification(notification=w133, notifier=w134) -> ()  [unwired: 1 in, 2 out]
          }
          event "Set Parameter", "Get Parameter": Value Change {
            n188 = event-data() -> ("CtlRef"=w172:refnum<vi>)  [unwired: 1 in]
            n189 = Get Notifier Status(notifier=w171) -> (notifier out=w166:refnum<notifier>, current notification=w169:T6)  [unwired: 1 in, 3 out]
            n190 = Bundle By Name(cluster=w169, "Running?"=FALSE) -> (w165:T6)
            n191 = property class="Bool"(reference=w172) -> ("Label.Text"=w170:string)  [unwired: 1 in, 2 out]
            n192 = Send Notification(notification=w165, notifier=w166) -> (notifier out=w164:refnum<notifier>)  [unwired: 1 in, 1 out]
            n193 = case shown="\"Set Parameter\"" w170 {
              tunnel: [Prime_Actions."Get Parameter" ("IDS Actions") Prime_Actions."Set Parameter" ("IDS Actions")] -> w161
              frame "Get Parameter", Default {
              }
              frame "Set Parameter" {
              }
            }
            n194 = for {
              N: 2000 -> [_]
              tunnel: w164 -> [w178]
              tunnel: [w177] -> w160
              tunnel: [w176] -> w163
              stop <- w174 stop-if-true
              n195 = Get Notifier Status(notifier=w178) -> (notifier out=w177:refnum<notifier>, current notification=w176:T6, # waiting=w175:i32)  [unwired: 1 in, 2 out]
              n196 = Wait (ms)(milliseconds to wait=u32 2) -> ()  [unwired: 1 out]
              n197 = Not Equal To 0?(x=w175) -> (x != 0?=w174:bool)
            }
            n198 = Bundle By Name(cluster=w163, "Prime Actions"=w161, "Prime Parameter"="Prime Parameter") -> (w159:T6)
            n199 = Send Notification(notification=w159, notifier=w160) -> (notifier out=w158:refnum<notifier>)  [unwired: 1 in, 1 out]
            n200 = Wait on Notification(notifier=w158, ignore previous (F)=TRUE) -> (notification=w156:T6)  [unwired: 2 in, 3 out]
            n201 = Unbundle By Name(w156) -> ("Prime Parameter"=w155:T2)
            n202 = local write "Prime Parameter"(w155) -> ()
          }
          event "Set ROI": Value Change {
            n203 = event-data() -> ("CtlRef"=w199:refnum<vi>)  [unwired: 1 in]
            n204 = Get Notifier Status(notifier=w198) -> (notifier out=w193:refnum<notifier>, current notification=w196:T6)  [unwired: 1 in, 3 out]
            n205 = Bundle By Name(cluster=w196, "Running?"=FALSE) -> (w192:T6)
            n206 = property class="Bool"(reference=w199) -> ("Label.Text"=w197:string)  [unwired: 1 in, 2 out]
            n207 = Send Notification(notification=w192, notifier=w193) -> (notifier out=w191:refnum<notifier>)  [unwired: 1 in, 1 out]
            n208 = case shown="\"Set ROI\"" w197 {
              tunnel: [Prime_Actions."Get ROI" ("IDS Actions") Prime_Actions."Set ROI" ("IDS Actions")] -> w189
              frame "Get ROI", Default {
              }
              frame "Set ROI" {
              }
            }
            n209 = for {
              N: 2000 -> [_]
              tunnel: w191 -> [w205]
              tunnel: [w204] -> w188
              tunnel: [w203] -> w190
              stop <- w201 stop-if-true
              n210 = Get Notifier Status(notifier=w205) -> (notifier out=w204:refnum<notifier>, current notification=w203:T6, # waiting=w202:i32)  [unwired: 1 in, 2 out]
              n211 = Wait (ms)(milliseconds to wait=u32 1) -> ()  [unwired: 1 out]
              n212 = Not Equal To 0?(x=w202) -> (x != 0?=w201:bool)
            }
            n213 = Bundle By Name(cluster=w190, "Prime Actions"=w189, "Prime ROI"="ROI Setup") -> (w187:T6)
            n214 = Send Notification(notification=w187, notifier=w188) -> (notifier out=w186:refnum<notifier>)  [unwired: 1 in, 1 out]
            n215 = Wait on Notification(notifier=w186, ignore previous (F)=TRUE) -> (notification=w184:T6)  [unwired: 2 in, 3 out]
            n216 = Unbundle By Name(w184) -> ("Prime ROI"=w183:T1)
            n217 = local write "ROI Setup"(w183) -> ()
          }
          event "# of Frames", "File Save Path": Value Change {
            n218 = event-data() -> ("CtlRef"=w216:refnum<vi>)  [unwired: 1 in]
            n219 = Get Notifier Status(notifier=w215) -> (notifier out=w213:refnum<notifier>, current notification=w212:T6)  [unwired: 1 in, 3 out]
            n220 = property class="Ctl"(reference=w216) -> ("Label.Text"=w214:string)  [unwired: 1 in, 2 out]
            n221 = case shown="\"# of Frames\", Default" w214 {
              tunnel: w213 -> [w220 w227]
              tunnel: w212 -> [w222 w226]
              tunnel: [w220 w227] -> w211
              tunnel: [w219 w225] -> w210
              tunnel: Prime_Actions."Error Check" ("IDS Actions") -> [w218 w223]
              frame "# of Frames", Default {
                n222 = Bundle By Name(cluster=w222, "# of frames"="# of Frames", "Prime Actions"=w218) -> (w219:T6)
              }
              frame "File Save Path" {
                n223 = Bundle By Name(cluster=w226, "File Path"="File Save Path", "Prime Actions"=w223) -> (w225:T6)
              }
            }
            n224 = Send Notification(notification=w210, notifier=w211) -> ()  [unwired: 1 in, 2 out]
          }
          event "Set Trigger": Value Change {
            n225 = event-data() -> ()  [unwired: 1 in, 1 out]
            n226 = Get Notifier Status(notifier=w232) -> (notifier out=w231:refnum<notifier>, current notification=w230:T6)  [unwired: 1 in, 3 out]
            n227 = Bundle By Name(cluster=w230, "Prime Actions"=Prime_Actions."Set Trigger") -> (w228:T6)
            n228 = Send Notification(notification=w228, notifier=w231) -> ()  [unwired: 1 in, 2 out]
          }
          event "Quit": Value Change {
            n229 = event-data() -> ("NewVal"=w234:bool)  [unwired: 1 in]
            n230 = Release Queue(queue=w240) -> ()  [unwired: 2 in, 3 out]
            n231 = Get Notifier Status(notifier=w239) -> (notifier out=w238:refnum<notifier>, current notification=w237:T6)  [unwired: 1 in, 3 out]
            n232 = Bundle By Name(cluster=w237, "Prime Actions"=Prime_Actions."Quit" ("IDS Actions")) -> (w235:T6)
            n233 = Send Notification(notification=w235, notifier=w238) -> ()  [unwired: 1 in, 2 out]
          }
        }
      }
      n234 = Release Notifier(notifier=w53, force destroy? (F)=TRUE) -> ()  [unwired: 1 in, 3 out]
    }
    frame Error {
      n235 = Release Notifier(notifier=w604, force destroy? (F)=TRUE, error in (no error)=w603) -> (error out=w592:errorcluster)  [unwired: 2 out]
      n236 = call <userlib>:"CameraClose.vi"("error in"=w592, "Camera Handle"=w593) -> ("error out"=w594:errorcluster)
      n237 = call <userlib>:"UninitToolkit.vi"("error in"=w594) -> ("error out"=w591:errorcluster)
      n238 = call "IMAQ Dispose"("Image"=w596, "error in (no error)"=w591) -> ("error out"=w595:errorcluster)  [unwired: 4 in]
      n239 = Unbundle By Name(w595) -> ("source"=w597:string)
      n240 = call <vilib>:"Space Constant.vi"() -> ("String"=w600:string)
      n241 = Concatenate Strings(w602, w600, "Device Error." ("string"), "\r", w597) -> (w601:string)
      n242 = One Button Dialog(message=w601) -> ()  [unwired: 1 in, 1 out]
    }
  }
